vi "red_but.vi"() -> ()   [LabVIEW 2021]
uses:
  conditions.ctl
  <vilib>/numeric/Random Number (Range) U64.vi
  <vilib>/numeric/sub_Random U32.vi
panel:
  out "notification 2":string="let's fight together!!! (with USA :))"
  out "problems":dbl(knob) scale=0.0..100.0
  in  "stop":bool
  out "leds":cluster{"1":bool, "2":bool, "3":bool}
  in  "bups":cluster{"bup1":bool, "bup2":bool, "bup3":bool}
  out "condition":T1
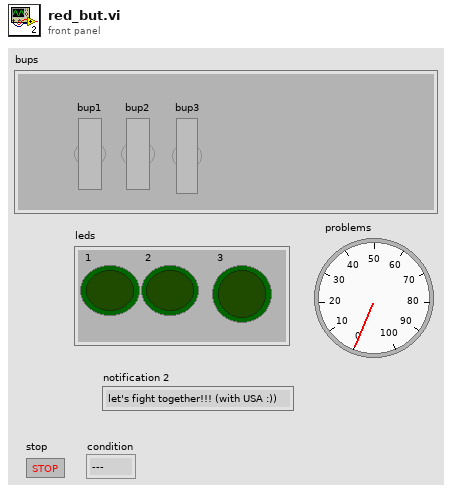
[diagram p1: front panel]
types:
  T1 = typedef "conditions.ctl" = enum16{"---", "0--", "00-", "000", "problems"}
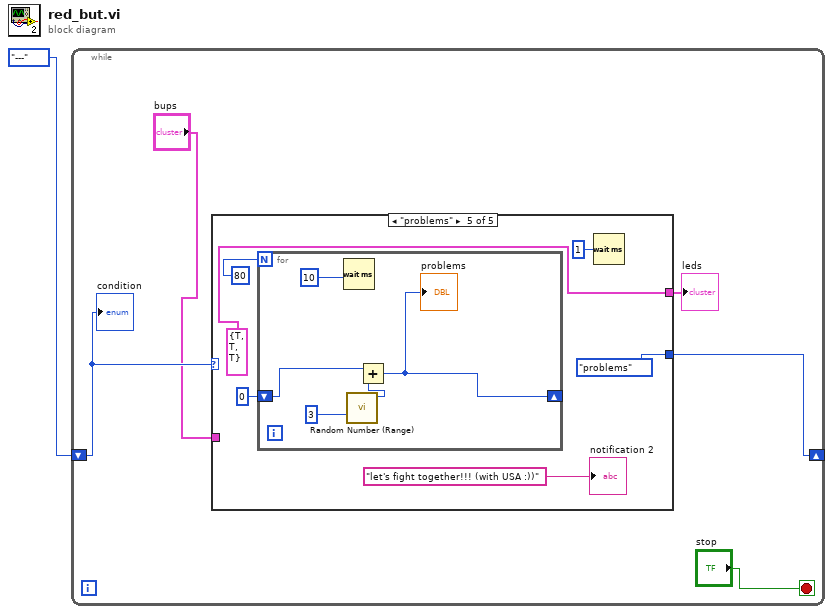
[diagram p0: block diagram]
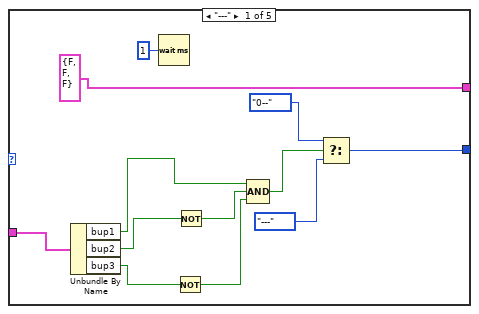
[diagram p2: hidden frame]
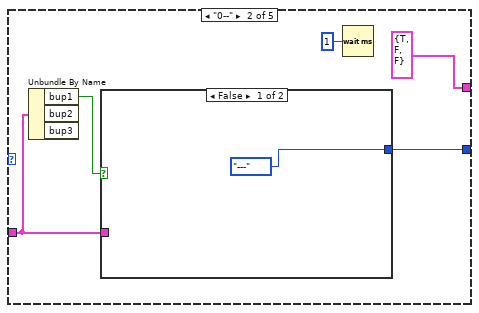
[diagram p3: hidden frame]
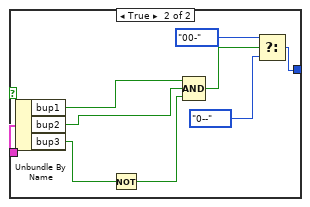
[diagram p4: hidden frame]
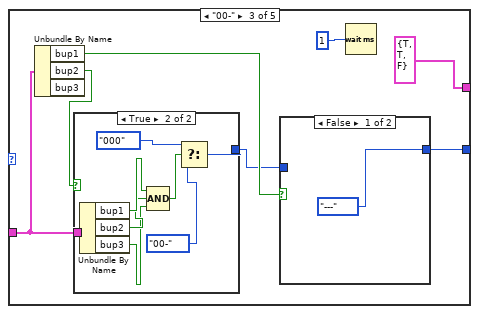
[diagram p5: hidden frame]
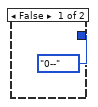
[diagram p7: hidden frame]
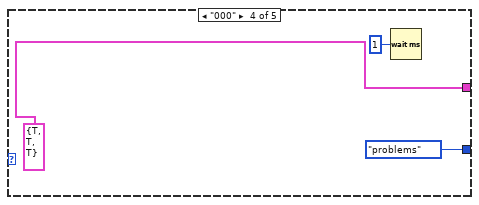
[diagram p8: hidden frame]
diagram:
  n1 = while {
    shift-right: [w5] -> _
    shift-left: conditions."---" ("conditions") -> [w6]
    stop <- "stop" stop-if-true
    n2 = case shown="\"problems\"" w6 {
      tunnel: [w12 w22 w35 conditions."problems" ("conditions") conditions."problems" ("conditions")] -> w5
      tunnel: "bups" -> [w11 w20 w37 _ _]
      tunnel: [cluster{"1":bool, "2":bool, "3":bool} {"1"=FALSE, "2"=FALSE, "3"=FALSE} ("leds") cluster{"1":bool, "2":bool, "3":bool} {"1"=TRUE, "2"=FALSE, "3"=FALSE} ("leds") cluster{"1":bool, "2":bool, "3":bool} {"1"=TRUE, "2"=TRUE, "3"=FALSE} ("leds") cluster{"1":bool, "2":bool, "3":bool} {"1"=TRUE, "2"=TRUE, "3"=TRUE} ("leds") cluster{"1":bool, "2":bool, "3":bool} {"1"=TRUE, "2"=TRUE, "3"=TRUE} ("leds")] -> w3
      frame "---" {
        n3 = Unbundle By Name(w11) -> ("bup1"=w10:bool, "bup2"=w9:bool, "bup3"=w8:bool)
        n4 = Wait (ms)(milliseconds to wait=u32 1) -> ()  [unwired: 1 out]
        n5 = Not(x=w8) -> (.not. x?=w17:bool)
        n6 = Not(x=w9) -> (.not. x?=w18:bool)
        n7 = Compound Arithmetic op=AND(w10, w18, w17) -> (w16:bool)
        n8 = Select(t=conditions."0--" ("conditions"), s=w16, f=conditions."---" ("conditions")) -> (s? t:f=w12:T1)
      }
      frame "0--" {
        n9 = Unbundle By Name(w20) -> ("bup1"=w19:bool)  [unwired: 2 out]
        n10 = case shown="False" w19 {
          tunnel: [conditions."---" ("conditions") w29] -> w22
          tunnel: w20 -> [_ w28]
          frame False {
          }
          frame True {
            n11 = Unbundle By Name(w28) -> ("bup1"=w27:bool, "bup2"=w25:bool, "bup3"=w26:bool)
            n12 = Not(x=w26) -> (.not. x?=w33:bool)
            n13 = Compound Arithmetic op=AND(w27, w25, w33) -> (w32:bool)
            n14 = Select(t=conditions."00-" ("conditions"), s=w32, f=conditions."0--" ("conditions")) -> (s? t:f=w29:T1)
          }
        }
        n15 = Wait (ms)(milliseconds to wait=u32 1) -> ()  [unwired: 1 out]
      }
      frame "00-" {
        n16 = Unbundle By Name(w37) -> ("bup1"=w36:bool, "bup2"=w38:bool)  [unwired: 1 out]
        n17 = case shown="True" w38 {
          tunnel: [conditions."0--" ("conditions") w48] -> w34
          tunnel: w37 -> [_ w47]
          frame False {
          }
          frame True {
            n18 = Unbundle By Name(w47) -> ("bup1"=w46:bool, "bup2"=w45:bool, "bup3"=w44:bool)
            n19 = Compound Arithmetic op=AND(w46, w45, w44) -> (w51:bool)
            n20 = Select(t=conditions."000" ("conditions"), s=w51, f=conditions."00-" ("conditions")) -> (s? t:f=w48:T1)
          }
        }
        n21 = case shown="False" w36 {
          tunnel: [conditions."---" ("conditions") w42] -> w35
          tunnel: w34 -> [_ w42]
          frame False {
          }
          frame True {
          }
        }
        n22 = Wait (ms)(milliseconds to wait=u32 1) -> ()  [unwired: 1 out]
      }
      frame "000" {
        n23 = Wait (ms)(milliseconds to wait=u32 1) -> ()  [unwired: 1 out]
      }
      frame "problems" {
        n24 = for {
          N: 80 -> [_]
          shift-right: [w61] -> _
          shift-left: u64 0 -> [w64]
          n25 = Wait (ms)(milliseconds to wait=u32 10) -> ()  [unwired: 1 out]
          n26 = call-poly <vilib>:"Random Number (Range).vi"("upper bound (100)"=u64 3) -> ("number"=w63:u64)  [unwired: 10 in]
          n27 = Add(x=w64, y=w63) -> (x+y=w61:u64)
          "problems" <- w61
        }
        n28 = Wait (ms)(milliseconds to wait=u32 1) -> ()  [unwired: 1 out]
        "notification 2" <- "let's fight together!!! (with USA :))"
      }
    }
    "leds" <- w3
    "condition" <- w6
  }
